vi "Draw All Legends.vi"(8 "error in (no error)":errorcluster caption="错误输入（无错误）", 10 "origin":cluster{"x":i16, "y":i16} caption="Origin", 11 "Gradient PieChart 输入":refnum<class "Gradient PieChart.lvclass"> caption="DNL_LabVIEW Object in") -> (0 "error out":errorcluster caption="错误输出", 3 "Gradient PieChart 输出":refnum<class "Gradient PieChart.lvclass"> caption="DNL_LabVIEW Object out")   [LabVIEW 2012, in "Gradient PieChart.lvclass"]
uses:
  Gradient PieChart.lvclass
  Gradient PieChart.lvclass/Gradient PieChart.ctl
  Legend Info.ctl
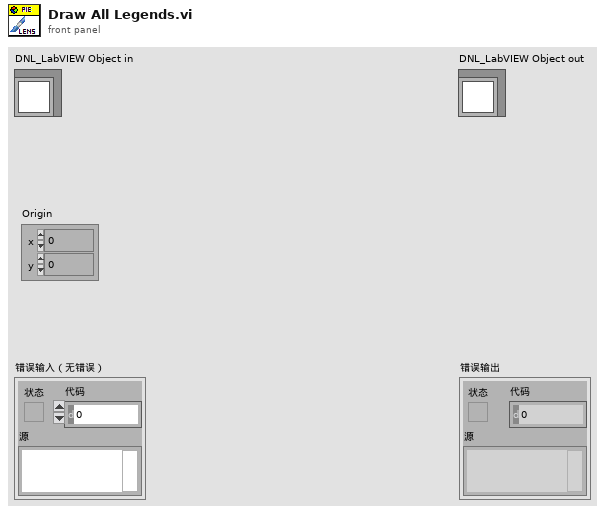
[diagram p1: front panel]
types:
  T1 = typedef "Gradient PieChart.lvclass/Legend Info.ctl" = cluster{"Name":string, "Percent":dbl, "TxtColor":u32, "Hor Space":i16, "Ver Space":i16, "Color Segement":u32[]}
  T2 = typedef "Gradient PieChart.lvclass/Info.ctl" = cluster{"Value":dbl, "Name":string, "NameTxtColor":u32, "Color Segement":u32[]}
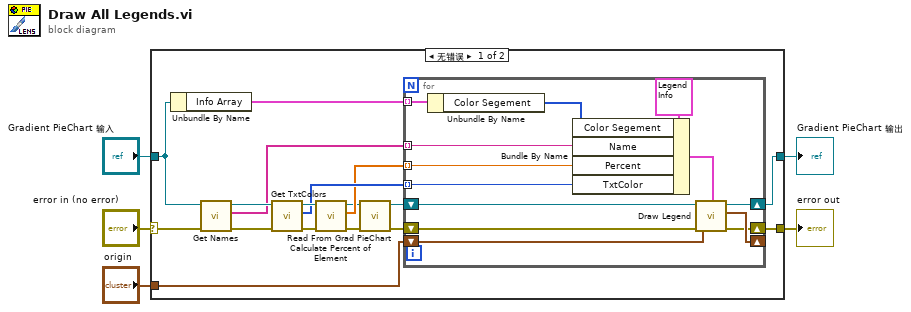
[diagram p0: block diagram]
diagram:
  n1 = case shown="无错误" "error in (no error)" {
    selector: "error in (no error)" -> [w22 w37]
    tunnel: [w7 w37] -> w4
    tunnel: [w6 w36] -> w2
    tunnel: "Gradient PieChart 输入" -> [w12 w36]
    tunnel: "origin" -> [w9 _]
    frame No Error {
      n2 = Unbundle By Name(w12) -> ("Info Array"=w11:T2[])
      n3 = call "Get Names.vi"("error in (no error)"=w22, "Gradient PieChart 输入"=w12) -> ("error out"=w20:errorcluster, "Names"=w17:string[], "Gradient PieChart 输出"=w21:refnum<class "Gradient PieChart.lvclass">)  [unwired: 7 in]
      n4 = call "Get TxtColors.vi"("error in (no error)"=w20, "Gradient PieChart 输入"=w21) -> ("error out"=w18:errorcluster, "NameTxtColor Array"=w16:u32[], "Gradient PieChart 输出"=w19:refnum<class "Gradient PieChart.lvclass">)  [unwired: 7 in]
      n5 = call "Calculate Percent of Element.vi"("error in (no error)"=w18, "Gradient PieChart 输入"=w19) -> ("error out"=w13:errorcluster, "Percent"=w15:dbl[], "Gradient PieChart 输出"=w14:refnum<class "Gradient PieChart.lvclass">)  [unwired: 6 in, 1 out]
      n6 = call "Read From Grad PieChart.vi"("error in (no error)"=w13, "Gradient PieChart输入"=w14) -> ("error out"=w8:errorcluster, "Gradient PieChart输出"=w10:refnum<class "Gradient PieChart.lvclass">)  [unwired: 7 in, 1 out]
      n7 = for {
        tunnel: w17 -> [w23] mode=indexing
        tunnel: w16 -> [w33] mode=indexing
        tunnel: w15 -> [w34] mode=indexing
        tunnel: w11 -> [w32] mode=indexing
        shift-right: [w30] -> w6
        shift-left: w10 -> [w31]
        shift-right: [w28] -> _
        shift-left: w9 -> [w29]
        shift-right: [w25] -> w7
        shift-left: w8 -> [w26]
        n8 = Unbundle By Name(w32) -> ("Color Segement"=w24:u32[])
        n9 = Bundle By Name(cluster=T1 {"Name"="", "Percent"=0.0, "TxtColor"=0, "Hor Space"=10, "Ver Space"=5, "Color Segement"=[16448250, 0, 16736786, 1198079]} ("Legend Info"), "Color Segement"=w24, "Name"=w23, "Percent"=w34, "TxtColor"=w33) -> (w27:T1)
        n10 = call "Draw Legend.vi"("error in (no error)"=w26, "Legend Info"=w27, "origin"=w29, "Gradient PieChart 输入"=w31) -> ("error out"=w25:errorcluster, "Next Origin"=w28:cluster{"x":i16, "y":i16}, "Gradient PieChart 输出"=w30:refnum<class "Gradient PieChart.lvclass">)  [unwired: 5 in]
      }
    }
    frame Error {
    }
  }
  "error out" <- w4
  "Gradient PieChart 输出" <- w2
